vi "Populate MC List Box.vi"(7 "Listbox Ref":refnum<vi>, 8 "Error In":errorcluster, 11 "Dependecy Config":T1) -> (0 "Error Out":errorcluster, 3 "Dependecy Config":T1)   [LabVIEW 2011, in "LMH-Toolbox.lvlib" / "LMH-Installer Tools.lvlib"]
uses:
  LMH-Installer Tools.lvlib
  Type Defs/Dependency Config.ctl
  Type Defs/Dependecy.ctl
  Common/Private/Web/Type Defs/Download Task.ctl
  Common/LMH-Common.lvlib
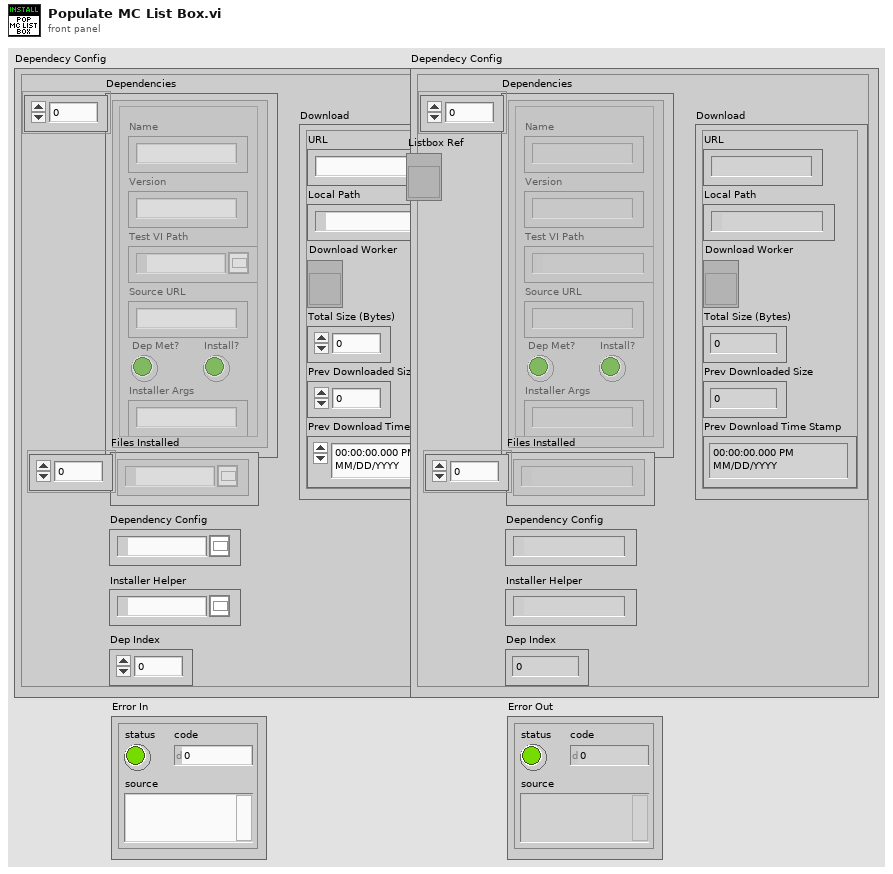
[diagram p1: front panel]
types:
  T1 = typedef "LMH-Toolbox.lvlib/LMH-Installer Tools.lvlib/Dependency Config.ctl" = cluster{"Dependencies":T2[], "Files Installed":path[], "Dependency Config":path, "Installer Helper":path, "Dep Index":i32, "Download":T3}
  T2 = typedef "LMH-Toolbox.lvlib/LMH-Installer Tools.lvlib/Dependecy.ctl" = cluster{"Name":string, "Version":string, "Test VI Path":path, "Source URL":string, "Dep Met?":bool, "Install?":bool, "Installer Args":string}
  T3 = typedef "LMH-Toolbox.lvlib/LMH-Common.lvlib/Download Task.ctl" = cluster{"URL":string, "Local Path":path, "Download Worker":refnum<vi>, "Total Size (Bytes)":u64, "Prev Downloaded Size":u64, "Prev Download Time Stamp":timestamp}
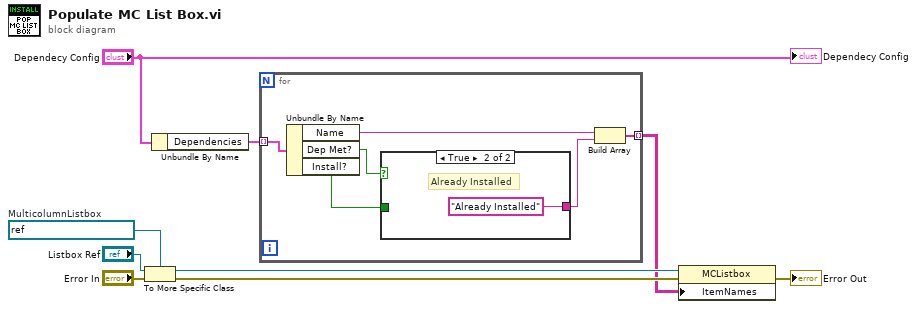
[diagram p0: block diagram]
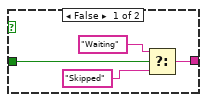
[diagram p2: hidden frame]
diagram:
  w5 = refnum<vi> refnum  # MulticolumnListbox
  n1 = To More Specific Class(target class=w5, reference="Listbox Ref", error in="Error In") -> (specific class reference=w3:refnum<vi>, error out=w4:errorcluster)
  n2 = Unbundle By Name("Dependecy Config") -> ("Dependencies"=w8:T2[])
  n3 = for {
    tunnel: w8 -> [w15] mode=indexing
    tunnel: [w10] -> w1 mode=indexing
    n4 = Unbundle By Name(w15) -> ("Name"=w12:string, "Dep Met?"=w14:bool, "Install?"=w11:bool)
    n5 = case shown="True" w14 {
      tunnel: [w19 "Already Installed"] -> w13
      tunnel: w11 -> [w18 _]
      frame False {
        n6 = Select(t="Waiting", s=w18, f="Skipped") -> (s? t:f=w19:string)
      }
      frame True {
        # "Already Installed"
      }
    }
    n7 = Build Array(w12, w13) -> (w10:string[])
  }
  n8 = property class="MCListbox"(reference=w3, error in=w4, "ItemNames"=w1) -> (error out=→"Error Out":errorcluster)  [unwired: 1 out]
  "Dependecy Config" <- "Dependecy Config"
